vi "lidar.vi"() -> ()   [LabVIEW 2015]
uses:
  <vilib>/Instr/_visa.llb/VISA Configure Serial Port (Instr).vi
panel:
  out "XY Graph":cluster{"Y":dbl[], "Y":dbl[]}[](graph) caption="Graphe XY"
  in  "timeout (10sec)":u32=10000 caption="timeout (10s)"
  out "chaîne du symbole 2":string
  out "chaîne du symbole":string
  in  "VISA resource name":refnum<visa-resource-name> caption="Nom de ressource VISA"
  in  "stop":bool
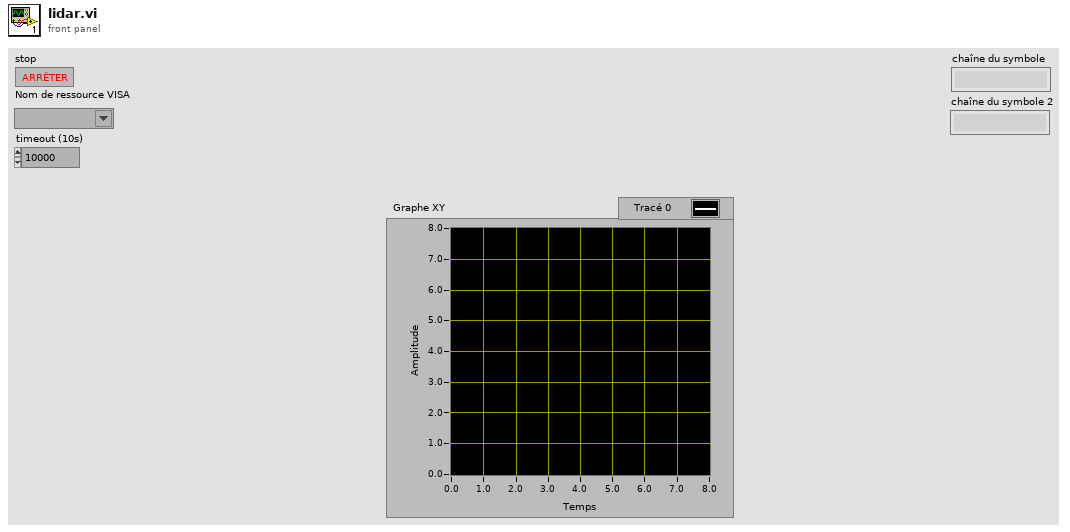
[diagram p1: front panel]
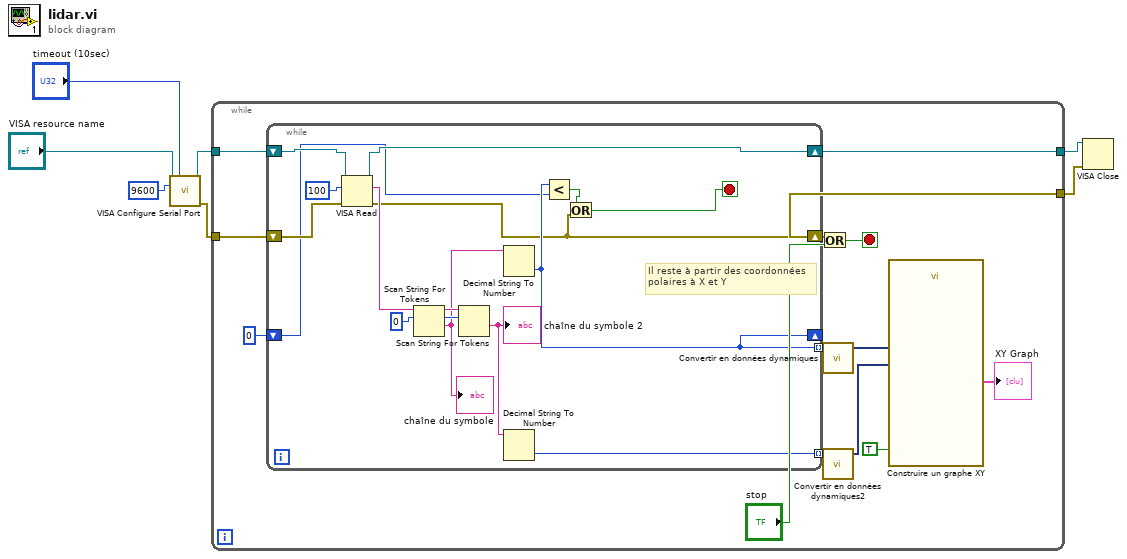
[diagram p0: block diagram]
diagram:
  n1 = call-poly "VISA Configure Serial Port"("VISA resource name"="VISA resource name", "timeout (10sec)"="timeout (10sec)", "baud rate (9600)"=u32 9600) -> ("VISA resource name out"=w5:refnum<visa-resource-name>, "error out"=w4:errorcluster)  [unwired: 11 in]
  n2 = while {
    tunnel: w5 -> [w20]
    tunnel: w4 -> [w19]
    tunnel: [w16] -> w3
    tunnel: [w15] -> w2
    stop <- w18 stop-if-true
    n3 = while {
      shift-right: [w34] -> w16
      shift-left: w20 -> [w36]
      shift-right: [w22] -> w15
      shift-left: w19 -> [w35]
      tunnel: [w25] -> w11 mode=indexing
      tunnel: [w26] -> w9 mode=indexing
      shift-right: [w25] -> _
      shift-left: 0 -> [w24]
      stop <- w21 stop-if-true
      # "Il reste à partir des coordonnées\npolaires à X et Y"
      n4 = VISA Read(VISA resource name=w36, byte count=u32 100 ("nombre d'octets"), error in (no error)=w35) -> (VISA resource name out=w34:refnum<visa-resource-name>, read buffer=w33:string, error out=w22:errorcluster)  [unwired: 1 out]
      n5 = Scan String For Tokens(8:0 ("offset"), 9:w33) -> (1:w28:string, 2:w30:i32, 3:w31:string)  [unwired: 4 in, 1 out]
      "chaîne du symbole" <- w28
      n6 = Scan String For Tokens(8:w30, 9:w31) -> (1:w27:string)  [unwired: 4 in, 3 out]
      "chaîne du symbole 2" <- w27
      n7 = Decimal String To Number(string=w28) -> (number=w25:i32)  [unwired: 2 in, 1 out]
      n8 = Decimal String To Number(string=w27) -> (number=w26:i32)  [unwired: 2 in, 1 out]
      n9 = Less?(x=w25, y=w24) -> (x < y?=w23:bool)
      n10 = Or(x=w23, y=w22) -> (x .or. y?=w21:bool)
    }
    n11 = Or(x=w15, y="stop") -> (x .or. y?=w18:bool)
    n12 = call "Convertir en données dynamiques"("Array"=w11) -> ("Dynamic Data Type"=w10:dynamicdata)  [unwired: 3 in]
    n13 = call "Convertir en données dynamiques2"("Array"=w9) -> ("Dynamic Data Type"=w8:dynamicdata)  [unwired: 3 in]
    n14 = call "Construire un graphe XY"("Reset"=TRUE, "Y Input"=w8, "X Input"=w10) -> ("XY Graph"=→"XY Graph":cluster{"X":dbl[], "Y":dbl[]}[])  [unwired: 7 in, 1 out]
  }
  n15 = VISA Close(VISA resource name=w3, error in (no error)=w2) -> ()  [unwired: 1 out]
